vi "TSC Material UI Theme Level--constant.vi"() -> (2 "UI theme levels":string[](array[string]))   [LabVIEW 2021]
doc: "This VI defines the constant value for the UI Theme Levels that are shown in the right click menu and are used in color application.\n\n\n<b>Code Developed By:</b>\nTechnology Service Corporation\n1983 S Liberty Drive\nBloomington, IN 47403\nwww.tsc.com/atcs\n\nDeveloper:\nDaniel Coons"
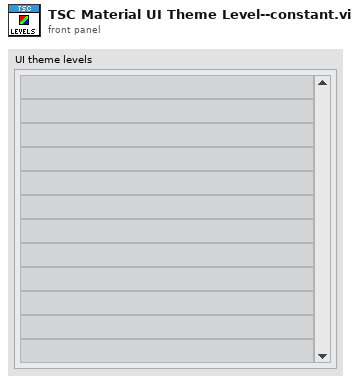
[diagram p1: front panel]
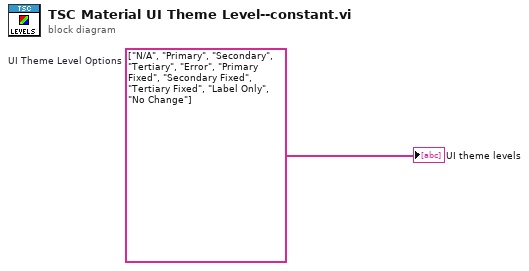
[diagram p0: block diagram]
diagram:
  w1 = string[] ["N/A", "Primary", "Secondary", "Tertiary", "Error", "Primary Fixed", "Secondary Fixed", "Tertiary Fixed", "Label Only", "No Change"]  # UI Theme Level Options
  "UI theme levels" <- w1
